vi "Utiltiysubs_PathPretreatment.vi"(11 "original trajectory":cluster{"x":dbl[], "y":dbl[]}) -> (3 "trajectory":T1)   [LabVIEW 2017]
uses:
  Trajectory.ctl
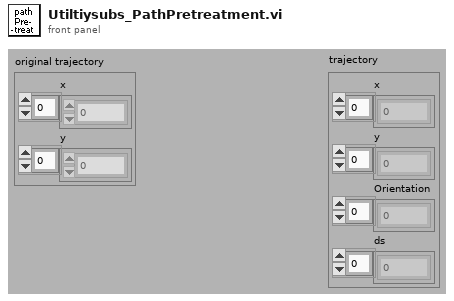
[diagram p1: front panel]
types:
  T1 = typedef "Trajectory.ctl" = cluster{"x":dbl[], "y":dbl[], "Orientation":dbl[], "ds":dbl[]}
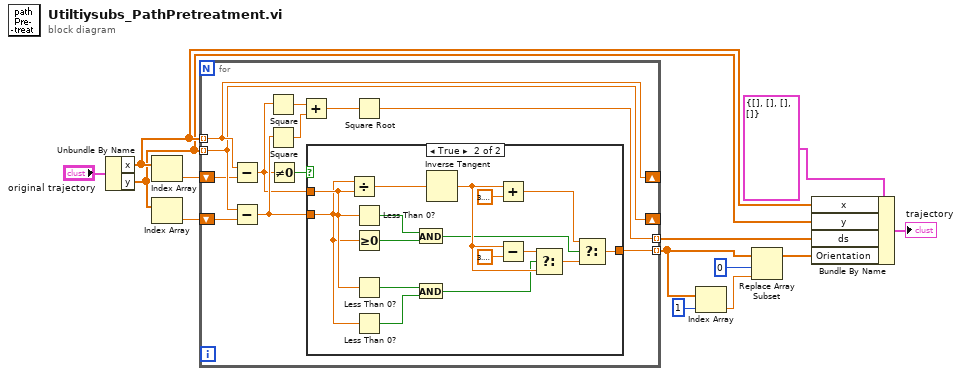
[diagram p0: block diagram]
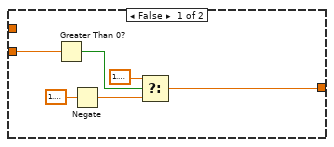
[diagram p2: hidden frame]
diagram:
  n1 = Unbundle By Name("original trajectory") -> ("x"=w10:dbl[], "y"=w7:dbl[])
  n2 = Index Array(array=w10) -> (element=w9:dbl)  [unwired: 1 in]
  n3 = Index Array(array=w7) -> (element=w8:dbl)  [unwired: 1 in]
  n4 = for {
    tunnel: w10 -> [w25] mode=indexing
    tunnel: w7 -> [w24] mode=indexing
    shift-right: [w25] -> _
    shift-left: w9 -> [w23]
    shift-right: [w24] -> _
    shift-left: w8 -> [w22]
    tunnel: [w21] -> w12 mode=indexing
    tunnel: [w20] -> w6 mode=indexing
    n5 = Subtract(x=w25, y=w23) -> (x-y=w14:dbl)
    n6 = Subtract(x=w24, y=w22) -> (x-y=w16:dbl)
    n7 = Square(x=w14) -> (x^2=w19:dbl)
    n8 = Square(x=w16) -> (x^2=w18:dbl)
    n9 = Not Equal To 0?(x=w14) -> (x != 0?=w15:bool)
    n10 = Add(x=w19, y=w18) -> (x+y=w17:dbl)
    n11 = case shown="True" w15 {
      tunnel: w16 -> [w31 w41]
      tunnel: w14 -> [_ w42]
      tunnel: [w30 w32] -> w20
      frame False {
        n12 = Greater Than 0?(x=w31) -> (x > 0?=w29:bool)
        n13 = Negate(x=1.5707963267948966) -> (-x=w26:dbl)
        n14 = Select(t=1.5707963267948966, s=w29, f=w26) -> (s? t:f=w30:dbl)
      }
      frame True {
        n15 = Divide(x=w41, y=w42) -> (x/y=w47:dbl)
        n16 = Less Than 0?(x=w42) -> (x < 0?=w37:bool)
        n17 = Greater Or Equal To 0?(x=w41) -> (x >= 0?=w38:bool)
        n18 = Less Than 0?(x=w42) -> (x < 0?=w44:bool)
        n19 = Less Than 0?(x=w41) -> (x < 0?=w43:bool)
        n20 = And(x=w37, y=w38) -> (x .and. y?=w36:bool)
        n21 = And(x=w44, y=w43) -> (x .and. y?=w39:bool)
        n22 = Inverse Tangent(1:w47) -> (0:w40:dbl)
        n23 = Add(x=w40, y=3.141592653589793) -> (x+y=w34:dbl)
        n24 = Subtract(x=w40, y=3.141592653589793) -> (x-y=w45:dbl)
        n25 = Select(t=w45, s=w39, f=w40) -> (s? t:f=w35:dbl)
        n26 = Select(t=w34, s=w36, f=w35) -> (s? t:f=w32:dbl)
      }
    }
    n27 = Square Root(x=w17) -> (sqrt(x)=w21:dbl)
  }
  n28 = Index Array(array=w6, index=1) -> (element=w3:dbl)
  n29 = Replace Array Subset(array=w6, new element=w3, index=0) -> (w5:dbl[])
  n30 = Bundle By Name(cluster=T1 {"x"=[], "y"=[], "Orientation"=[], "ds"=[]} ("trajectory"), "x"=w10, "y"=w7, "ds"=w12, "Orientation"=w5) -> (→"trajectory":T1)
